vi "set_clock_params.vi"(5 "duration high":dbl[unit], 6 "frequency":dbl[unit], 7 "offset":dbl[unit], 8 "error in (no error)":errorcluster, 9 "repetitions":i32, 10 "duty cycle":dbl[unit], 11 "Stimulator090724Scaffold in":refnum<class "Stimulator090724Scaffold.lvclass">) -> (0 "error out":errorcluster, 3 "Stimulator090724Scaffold out":refnum<class "Stimulator090724Scaffold.lvclass">)   [LabVIEW 2010, in "Stimulator090724Scaffold.lvclass"]
uses:
  Stimulator090724Scaffold.lvclass
  Stimulator090724Scaffold.lvclass/Stimulator090724Scaffold.ctl
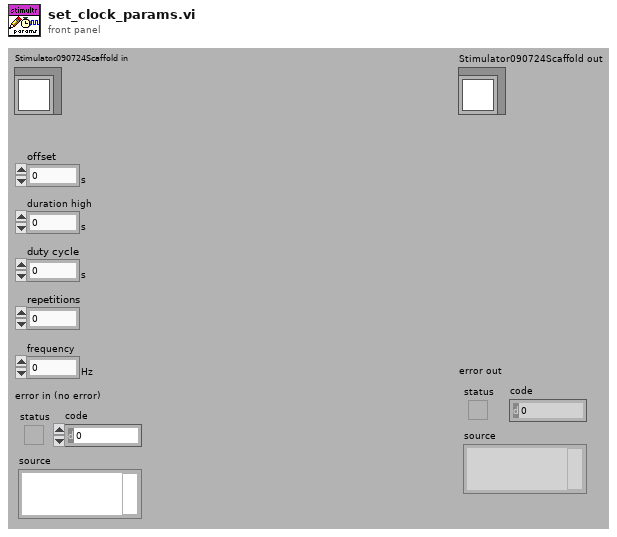
[diagram p1: front panel]
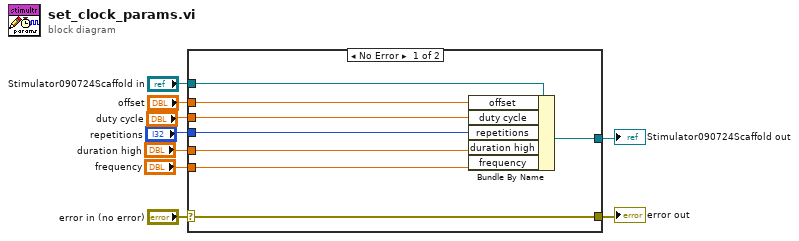
[diagram p0: block diagram]
diagram:
  n1 = case shown="No Error" "error in (no error)" {
    selector: "error in (no error)" -> [w11 w19]
    tunnel: [w11 w19] -> w8
    tunnel: [w16 w18] -> w6
    tunnel: "Stimulator090724Scaffold in" -> [w17 w18]
    tunnel: "duration high" -> [w12 _]
    tunnel: "offset" -> [w15 _]
    tunnel: "duty cycle" -> [w14 _]
    tunnel: "repetitions" -> [w13 _]
    tunnel: "frequency" -> [w10 _]
    frame No Error {
      n2 = Bundle By Name(cluster=w17, "offset"=w15, "duty cycle"=w14, "repetitions"=w13, "duration high"=w12, "frequency"=w10) -> (w16:refnum<class "Stimulator090724Scaffold.lvclass">)
    }
    frame Error {
    }
  }
  "error out" <- w8
  "Stimulator090724Scaffold out" <- w6
